vi "Motion@GoSafe__Parameter.vi"(1 "ParamterIn":string) -> (0 "ParamterOut":string)   [LabVIEW 2020]
panel:
  in  "Z=":string(combo)
  in  "PointName":string(combo)
  in  "Speed":string(combo)
  in  "MotorName":string(combo)
  in  "Confirm":bool
  # "Motion@GoSafe $Motor,$Speed,$Point,Z=XXX"
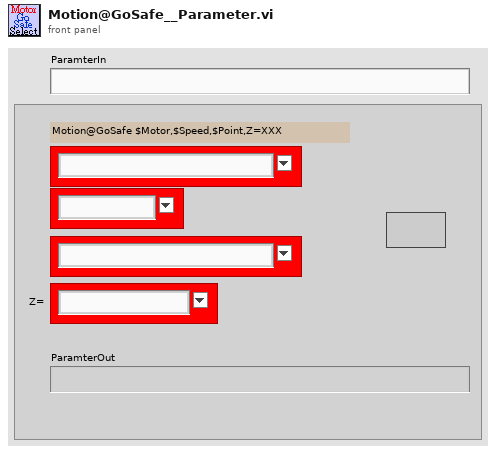
[diagram p1: front panel]
types:
  T1 = enum16{"Get", "UpdatePointS", "Init", "UpdateIndex", "GetCurrent&Index+1", "GetWithIndex", "ChkLast", "GetCurrent"}
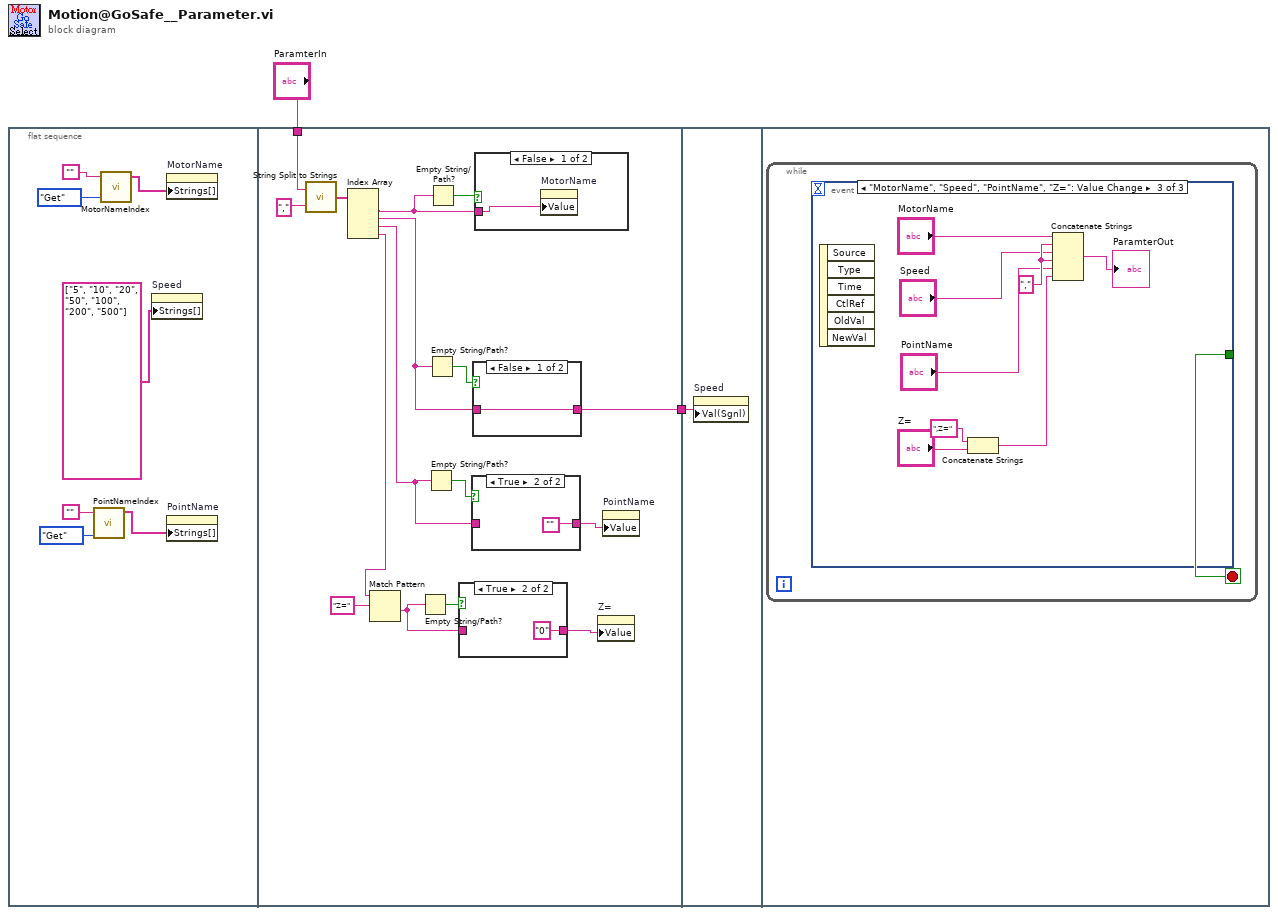
[diagram p0: block diagram]
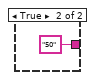
[diagram p4: hidden frame]
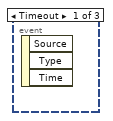
[diagram p6: hidden frame]
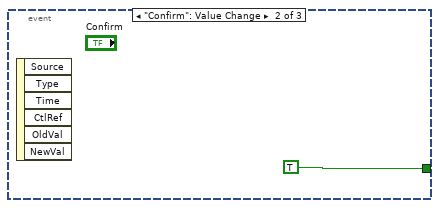
[diagram p7: hidden frame]
diagram:
  n1 = flat-sequence {
    tunnel: "ParamterIn" -> [w21]
    tunnel: [w16] -> w1
    tunnel: w1 -> [w33]
    frame #0 {
      n2 = call "PointNameIndex.vi"("OP"=T1."Get", "PointName"="") -> ("PointNameList"=w3:string[])  [unwired: 4 in, 5 out]
      n3 = call "MotorNameIndex.vi"("OP"=enum16{"Get", "Update", "Init"}."Get", "MotorName"="") -> ("MotorList"=w7:string[])  [unwired: 1 in, 2 out]
      n4 = property on="Speed" class="CmbBox"("Strings[]"=string[] ["5", "10", "20", "50", "100", "200", "500"] ("Strings []")) -> ()  [unwired: 2 in, 2 out]
      n5 = property on="MotorName" class="CmbBox"("Strings[]"=w7) -> ()  [unwired: 2 in, 2 out]
      n6 = property on="PointName" class="CmbBox"("Strings[]"=w3) -> ()  [unwired: 2 in, 2 out]
    }
    frame #1 {
      n7 = call "String Split to Strings.vi"("search string/char (-)"=",", "String"=w21) -> ("Array"=w23:string[])
      n8 = Index Array(array=w23) -> (element #1=w20:string, element #2=w19:string, element #3=w17:string, element #4=w14:string)  [unwired: 4 in]
      n9 = Match Pattern(string=w14, regular expression="Z=") -> (after substring=w11:string)  [unwired: 1 in, 3 out]
      n10 = Empty String/Path?(string/path=w11) -> (empty?=w12:bool)
      n11 = Empty String/Path?(string/path=w17) -> (empty?=w18:bool)
      n12 = Empty String/Path?(string/path=w19) -> (empty?=w24:bool)
      n13 = Empty String/Path?(string/path=w20) -> (empty?=w25:bool)
      n14 = case shown="True" w12 {
        tunnel: [w26 "0" ("ParamterIn")] -> w10
        tunnel: w11 -> [w26 _]
        frame False {
        }
        frame True {
        }
      }
      n15 = case shown="True" w18 {
        tunnel: [w28 ""] -> w15
        tunnel: w17 -> [w28 _]
        frame False {
        }
        frame True {
        }
      }
      n16 = case shown="False" w24 {
        tunnel: [w30 "50" ("ParamterIn")] -> w16
        tunnel: w19 -> [w30 _]
        frame False {
        }
        frame True {
        }
      }
      n17 = case shown="False" w25 {
        tunnel: w20 -> [w32 _]
        frame False {
          n18 = property on="MotorName" class="CmbBox"("Value"=w32) -> ()  [unwired: 2 in, 2 out]
        }
        frame True {
        }
      }
      n19 = property on="Z=" class="CmbBox"("Value"=w10) -> ()  [unwired: 2 in, 2 out]
      n20 = property on="PointName" class="CmbBox"("Value"=w15) -> ()  [unwired: 2 in, 2 out]
    }
    frame #2 {
      n21 = property on="Speed" class="CmbBox"("Val(Sgnl)"=w33) -> ()  [unwired: 2 in, 2 out]
    }
    frame #3 {
      n22 = while {
        stop <- w34 stop-if-true
        n23 = event shown="[2] \"MotorName\", \"Speed\", \"PointName\", \"Z=\": Value Change" {
          selector: _ -> [_ _ _]
          dyn-events: _ -> [_ _ _]
          timeout: _ -> [_ _ _]
          tunnel: [_ TRUE _] -> w34
          event Timeout {
            n24 = event-data() -> ()  [unwired: 1 in, 3 out]
          }
          event "Confirm": Value Change {
            n25 = event-data() -> ()  [unwired: 1 in, 6 out]
          }
          event "MotorName", "Speed", "PointName", "Z=": Value Change {
            w41 = "," ("string")
            n26 = event-data() -> ()  [unwired: 1 in, 6 out]
            n27 = Concatenate Strings(",Z=" ("string"), "Z=") -> (w36:string)
            n28 = Concatenate Strings("MotorName", w41, "Speed", w41, "PointName", w36) -> (→"ParamterOut":string)
          }
        }
      }
    }
  }
